vi "eDIDS-24XX-FPGA2-EPTx.vi"() -> ()   [LabVIEW 2015, in "ECS-FPGA.lvlib"]
uses:
  ECS-FPGA.lvlib
  <vilib>/Powertrain Controls/Device Drivers/Engine Position Tracking/EPTx/RevA/FPGA/Controls/EPTxTooth.ctl
  <vilib>/Powertrain Controls/Device Drivers/Engine Position Tracking/EPTx/RevA/FPGA/Controls/EPTxControl.ctl
  <vilib>/Powertrain Controls/Device Drivers/Engine Position Tracking/EPTx/RevA/FPGA/Controls/EPTxConfig.ctl
  <vilib>/Powertrain Controls/Device Drivers/Engine Position Tracking/EPTx/RevA/FPGA/Controls/EPTxSupervisor.ctl
  <vilib>/Powertrain Controls/Device Drivers/Engine Position Tracking/EPTx/RevA/FPGA/Controls/EPTxFuelSparkControl.ctl
  <vilib>/Platform/TimedLoop/XDataNode/timing_clust.ctl
  <vilib>/Platform/TimedLoop/XDataNode/nitl_modes.ctl
  <vilib>/Platform/TimedLoop/XDataNode/wakeup.ctl
  <vilib>/Powertrain Controls/Device Drivers/Engine Position Tracking/EPTx/RevA/FPGA/Controls/EPTxSignals.ctl
  <vilib>/rvi/Emulation/niFpgaSctlEmulationGetInTimedLoop.vi
  <vilib>/rvi/Emulation/niFpgaEmulationReportErrorSimple.vi
  <vilib>/rvi/Emulation/niFpgaGetClockAttributes.vi
  <vilib>/rvi/Emulation/niFpgaCriticalErrorInLSC.vi
  <vilib>/rvi/eio/common/nirviEmuTemplateMethod_errors.vi
  <vilib>/Platform/TimedLoop/XDataNode/XDataNode.xnode
  <vilib>/eio/EIONode/EIONode.xnode
  <vilib>/Platform/TimedLoop/XDataNode/XDNodeRunTimeDep.lvlib
  <vilib>/Powertrain Controls/Device Drivers/Engine Position Tracking/EPTx/RevA/FPGA/EPTx - RevA - FPGA.lvlib
panel:
  out "O2-1.Data":T1
  in  "O2-1.Control":T2
  in  "ESTTL-2.Sequences":T3(array[cluster])
  in  "ESTTL-2.Config":T4
  in  "ESTTL-1.Config":T4
  in  "ESTTL-1.Sequences":T3(array[cluster])
  in  "PFI-1.FuelControl 4":T5
  in  "PFI-1.FuelControl 3":T5
  in  "PFI-1.FuelControl 2":T5
  in  "PFI-1.FuelControl 1":T5
  out "PFI-1.Data":T6 caption="PFIData"
  in  "PFI-1.IPhaseInterface":T7(array[cluster])=[{"IPhaseCurrent"=0, "IPhaseDuration"=0}, {"IPhaseCurrent"=0, "IPhaseDuration"=0}, {"IPhaseCurrent"=0, "IPhaseDuration"=0}, {"IPhaseCurrent"=0, "IPhaseDuration"=0}, {"IPhaseCurrent"=0, "IPhaseDuration"=0}, {"IPhaseCurrent"=0, "IPhaseDuration"=0}, {"IPhaseCurrent"=0, "IPhaseDuration"=0}, {"IPhaseCurrent"=0, "IPhaseDuration"=0}] caption="IPhaseInterface"
  in  "PFI-1.LowsidePWM":T8 caption="LowsidePWM"
  in  "PFI-1.Control":T9 caption="PFIControl"
  in  "PFI-2.Control":T9 caption="PFIControl"
  in  "PFI-2.LowsidePWM":T8 caption="LowsidePWM"
  in  "PFI-2.IPhaseInterface":T7(array[cluster])=[{"IPhaseCurrent"=0, "IPhaseDuration"=0}, {"IPhaseCurrent"=0, "IPhaseDuration"=0}, {"IPhaseCurrent"=0, "IPhaseDuration"=0}, {"IPhaseCurrent"=0, "IPhaseDuration"=0}, {"IPhaseCurrent"=0, "IPhaseDuration"=0}, {"IPhaseCurrent"=0, "IPhaseDuration"=0}, {"IPhaseCurrent"=0, "IPhaseDuration"=0}, {"IPhaseCurrent"=0, "IPhaseDuration"=0}] caption="IPhaseInterface"
  out "PFI-2.Data":T6 caption="PFIData"
  in  "PFI-2.FuelControl 1":T5
  in  "PFI-2.FuelControl 2":T5
  in  "PFI-2.FuelControl 3":T5
  in  "PFI-2.FuelControl 4":T5
  in  "EPTx.Aux3":u8
  in  "EPTx.Primary":u8
  in  "EPTx.Aux1":u8
  out "EPTxSupervisor":T10
  in  "EPTxConfig":T11
  in  "EPTxControl":T12
  out "EPTxTooth":T13
  in  "EPTx.Aux2":u8
  in  "EPTx.Aux4":u8
  out "VRHall-1.DigitalTriggers":u32
  out "Throttle-1.Data":T14 caption="ThrottleData"
  in  "Throttle-1.Control":T15 caption="ThrottleControl"
  out "9411-3.5.PPWData":T16
  out "9411-3.4.PPWData":T16
  out "9411-3.3.PPWData":T16
  out "9411-3.2.PPWData":T16
  out "9411-3.1.PPWData":T16
  out "9411-3.0.PPWData":T16
  in  "9411-3.0.Filt":u16
  in  "9411-3.1.Filt":u16
  in  "9411-3.2.Filt":u16
  in  "9411-3.3.Filt":u16
  in  "9411-3.4.Filt":u16
  in  "9411-3.5.Filt":u16
  in  "9411-3.Invert":u8
  out "9411-3.DigitalTriggers":u32
  out "VRHall-1.6.PPWData":T16
  out "VRHall-1.5.PPWData":T16
  out "VRHall-1.4.PPWData":T16
  out "VRHall-1.3.PPWData":T16
  out "VRHall-1.2.PPWData":T16
  out "VRHall-1.1.PPWData":T16
  in  "VRHall-1.Invert":u8
  in  "VRHall-1.5.Filt":u16
  in  "VRHall-1.4.Filt":u16
  in  "VRHall-1.3.Filt":u16
  in  "VRHall-1.2.Filt":u16
  in  "VRHall-1.1.Filt":u16
  in  "VRHall-1.6.Filt":u16
  out "VRHall-1.Data":T17 caption="VrHallData"
  in  "VRHall-1.Control":T18 caption="VrHallControl"
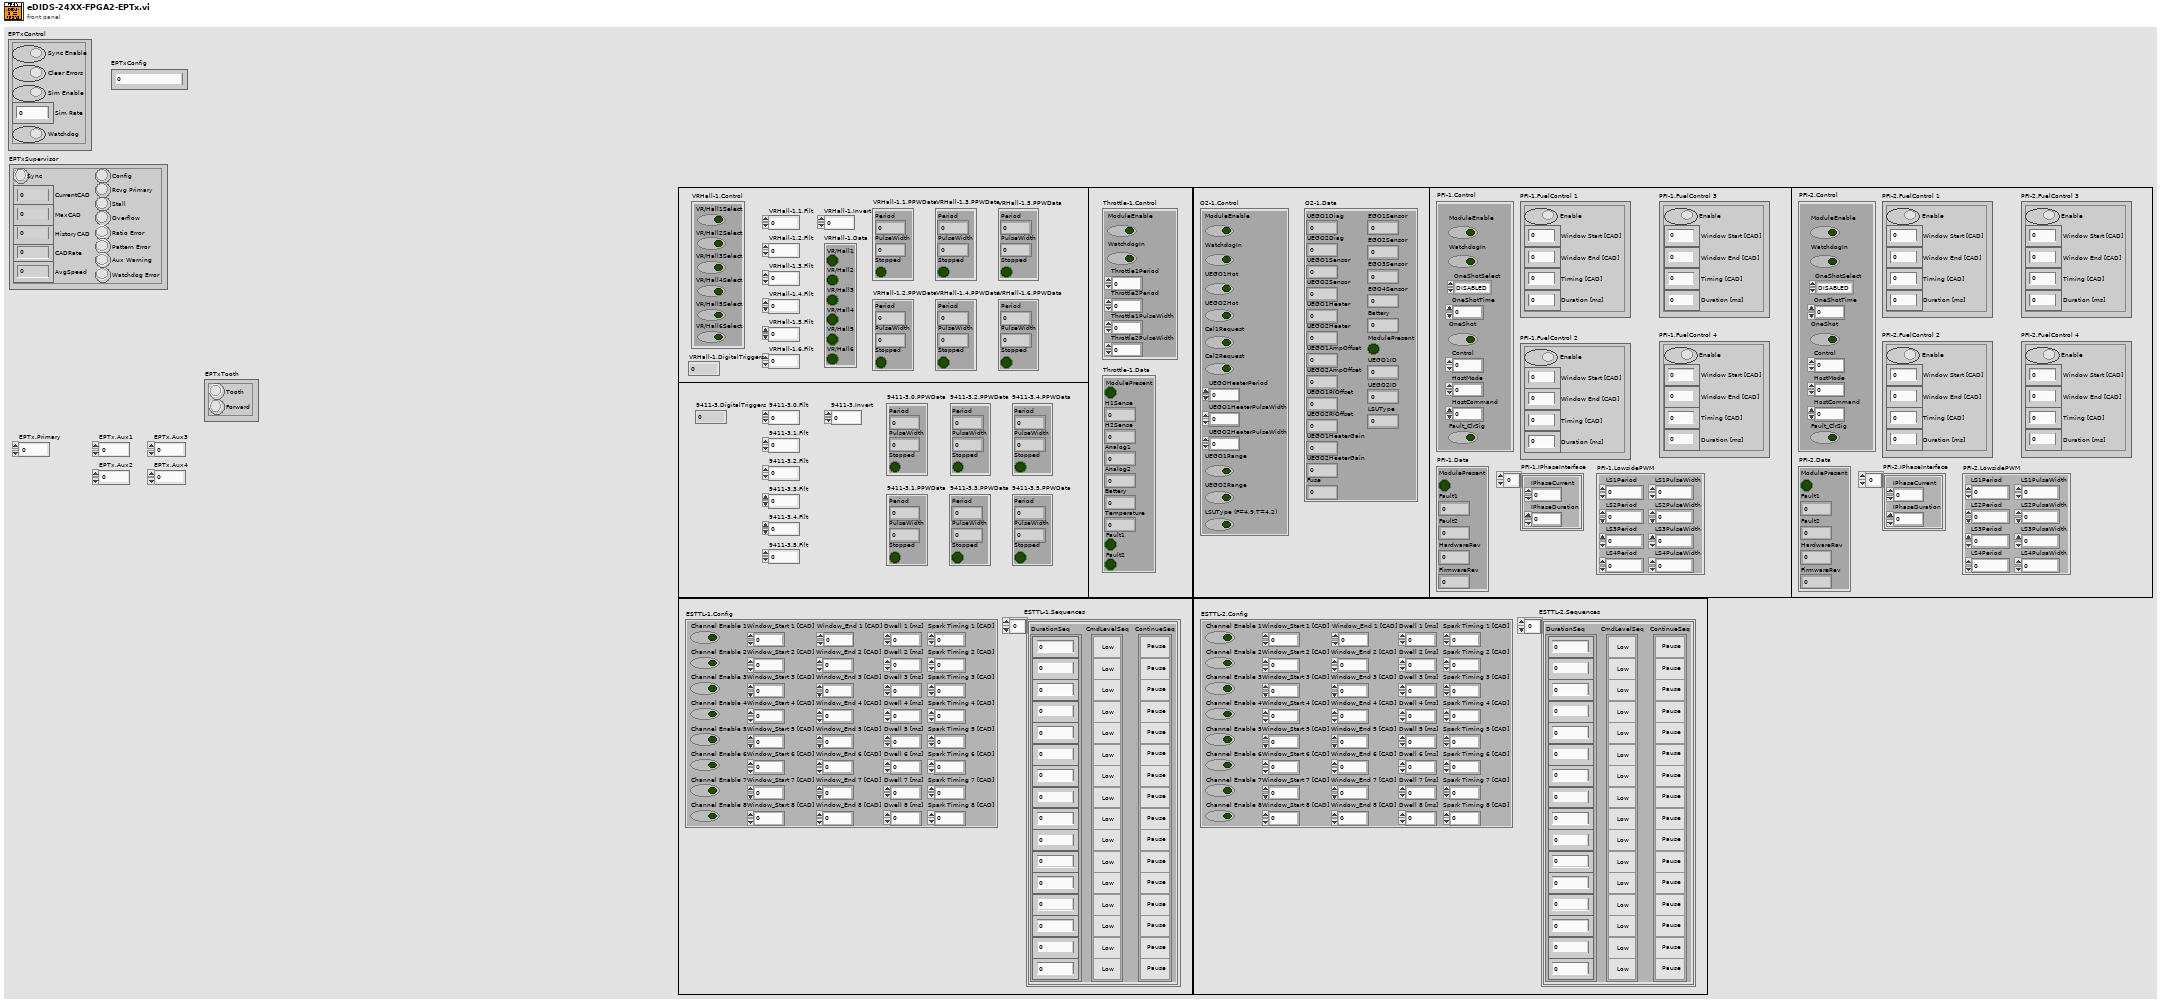
[diagram p1: front panel]
types:
  T1 = cluster{"UEGO1Diag":u8, "UEGO2Diag":u8, "UEGO1Sensor":u16, "UEGO2Sensor":u16, "UEGO1Heater":u16, "UEGO2Heater":u16, "UEGO1AmpOffset":u16, "UEGO2AmpOffset":u16, "UEGO1RIOffset":u16, "UEGO2RIOffset":u16, "UEGO1HeaterGain":u16, "UEGO2HeaterGain":u16, "Fuse":u16, "EGO1Sensor":u16, "EGO2Sensor":u16, "EGO3Sensor":u16, "EGO4Sensor":u16, "Battery":u16, "ModulePresent":bool, "UEGO1ID":u8, "UEGO2ID":u8, "LSUType":u8}
  T2 = cluster{"ModuleEnable":bool, "WatchdogIn":bool, "UEGO1Hot":bool, "UEGO2Hot":bool, "Cal1Request":bool, "Cal2Request":bool, "UEGOHeaterPeriod":u16, "UEGO1HeaterPulseWidth":u16, "UEGO2HeaterPulseWidth":u16, "UEGO1Range":bool, "UEGO2Range":bool, "LSUType (F=4.9,T=4.2)":bool}
  T3 = cluster{"DurationSeq":u32[], "CmdLevelSeq":bool[], "ContinueSeq":bool[]}[]
  T4 = cluster{"Channel Enable 1":bool, "Window_Start 1 [CAD]":fxp<+,18,11>, "Window_End 1 [CAD]":fxp<+,18,11>, "Dwell 1 [ms]":fxp<+/-,22,9>, "Spark Timing 1 [CAD]":fxp<+,18,11>, "Channel Enable 2":bool, "Window_Start 2 [CAD]":fxp<+,18,11>, "Window_End 2 [CAD]":fxp<+,18,11>, "Dwell 2 [ms]":fxp<+/-,22,9>, "Spark Timing 2 [CAD]":fxp<+,18,11>, "Channel Enable 3":bool, "Window_Start 3 [CAD]":fxp<+,18,11>, "Window_End 3 [CAD]":fxp<+,18,11>, "Dwell 3 [ms]":fxp<+/-,22,9>, "Spark Timing 3 [CAD]":fxp<+,18,11>, "Channel Enable 4":bool, "Window_Start 4 [CAD]":fxp<+,18,11>, "Window_End 4 [CAD]":fxp<+,18,11>, "Dwell 4 [ms]":fxp<+/-,22,9>, "Spark Timing 4 [CAD]":fxp<+,18,11>, "Channel Enable 5":bool, "Window_Start 5 [CAD]":fxp<+,18,11>, "Window_End 5 [CAD]":fxp<+,18,11>, "Dwell 5 [ms]":fxp<+/-,22,9>, "Spark Timing 5 [CAD]":fxp<+,18,11>, "Channel Enable 6":bool, "Window_Start 6 [CAD]":fxp<+,18,11>, "Window_End 6 [CAD]":fxp<+,18,11>, "Dwell 6 [ms]":fxp<+/-,22,9>, "Spark Timing 6 [CAD]":fxp<+,18,11>, "Channel Enable 7":bool, "Window_Start 7 [CAD]":fxp<+,18,11>, "Window_End 7 [CAD]":fxp<+,18,11>, "Dwell 7 [ms]":fxp<+/-,22,9>, "Spark Timing 7 [CAD]":fxp<+,18,11>, "Channel Enable 8":bool, "Window_Start 8 [CAD]":fxp<+,18,11>, "Window_End 8 [CAD]":fxp<+,18,11>, "Dwell 8 [ms]":fxp<+/-,22,9>, "Spark Timing 8 [CAD]":fxp<+,18,11>}
  T5 = typedef "EPTx - RevA - FPGA.lvlib/EPTxFuelSparkControl.ctl" = cluster{"Enable":bool, "Window Start [CAD]":fxp<+,18,11>, "Window End [CAD]":fxp<+,18,11>, "Timing [CAD]":fxp<+,18,11>, "Duration [ms]":fxp<+/-,22,9>}
  T6 = cluster{"ModulePresent":bool, "Fault1":u8, "Fault2":u8, "HardwareRev":u8, "FirmwareRev":u8}
  T7 = cluster{"IPhaseCurrent":u16, "IPhaseDuration":u16}[]
  T8 = cluster{"LS1Period":u32, "LS1PulseWidth":u32, "LS2Period":u32, "LS2PulseWidth":u32, "LS3Period":u32, "LS3PulseWidth":u32, "LS4Period":u32, "LS4PulseWidth":u32}
  T9 = cluster{"ModuleEnable":bool, "WatchdogIn":bool, "OneShotSelect":enum8{"DISABLED", "PFI 1", "PFI 2", "PFI 3", "PFI 4"}, "OneShotTime":u32, "OneShot":bool, "Control":u16, "HostMode":u8, "HostCommand":u32, "Fault_ClrSig":bool}
  T10 = typedef "EPTx - RevA - FPGA.lvlib/EPTxSupervisor.ctl" = cluster{"Sync":bool, "CurrentCAD":fxp<+,18,11>, "MaxCAD":fxp<+,11,11>, "HistoryCAD":fxp<+,11,11>, "CADRate":fxp<+,22,8>, "AvgSpeed":fxp<+,17,15>, "Config":bool, "Rcvg Primary":bool, "Stall":bool, "Overflow":bool, "Ratio Error":bool, "Pattern Error":bool, "Aux Warning":bool, "Watchdog Error":bool}
  T11 = typedef "EPTx - RevA - FPGA.lvlib/EPTxConfig.ctl" = u64
  T12 = typedef "EPTx - RevA - FPGA.lvlib/EPTxControl.ctl" = cluster{"Sync Enable":bool, "Clear Errors":bool, "Sim Enable":bool, "Sim Rate":fxp<+,24,6>, "Watchdog":bool}
  T13 = typedef "EPTx - RevA - FPGA.lvlib/EPTxTooth.ctl" = cluster{"Tooth":bool, "Forward":bool}
  T14 = cluster{"ModulePresent":bool, "H1Sense":i16, "H2Sense":i16, "Analog1":i16, "Analog2":i16, "Battery":i16, "Temperature":i16, "Fault1":bool, "Fault2":bool}
  T15 = cluster{"ModuleEnable":bool, "WatchdogIn":bool, "Throttle1Period":u16, "Throttle2Period":u16, "Throttle1PulseWidth":i16, "Throttle2PulseWidth":i16}
  T16 = cluster{"Period":u32, "PulseWidth":u32, "Stopped":bool}
  T17 = cluster{"VR/Hall1":bool, "VR/Hall2":bool, "VR/Hall3":bool, "VR/Hall4":bool, "VR/Hall5":bool, "VR/Hall6":bool}
  T18 = cluster{"VR/Hall1Select":bool, "VR/Hall2Select":bool, "VR/Hall3Select":bool, "VR/Hall4Select":bool, "VR/Hall5Select":bool, "VR/Hall6Select":bool}
  T19 = typedef "XDNodeRunTimeDep.lvlib/timing_clust.ctl" = cluster{"Expected End [f-1]":u64, "Actual End [f-1]":u64, "Finished Late? [f-1]":bool, "Expected End [i-1]":u64, "Actual End [i-1]":u64, "Finished Late? [i-1]":bool, "Expected Start [i]":u64, "Actual Start [i]":u64, "Expected Start [f]":u64, "Actual Start [f]":u64, "Source Name":string, "Structure Name":string, "Period":i64, "Deadline":i64, "Offset":i64, "Start":i64, "Priority":i32, "Timeout":i32, "Mode":T20, "Wakeup Reason":T21, "Error":errorcluster, "Source Type":string, "Secondary Source Type":string, "Global End Time":u64, "Global Start Time":u64, "Frame Duration":u64, "Iteration Duration":u64, "Assigned CPU":i32, "I/O Scan Engine Mode":u32}
  T20 = typedef "XDNodeRunTimeDep.lvlib/nitl_modes.ctl" = enum32{"No Change", "Process missed periods, maintain original phase", "Discard missed periods, maintain original phase", "Process missed periods, ignore original phase", "Discard missed periods, ignore original phase"}
  T21 = typedef "XDNodeRunTimeDep.lvlib/wakeup.ctl" = enum32{"Normal", "Aborted", "Asynchronous wakeup", "Timing source error", "Timed loop error", "Timeout"}
  T22 = typedef "EPTx - RevA - FPGA.lvlib/EPTxSignals.ctl" = cluster{"Primary":bool, "Aux 1":bool, "Aux 2":bool, "Aux 3":bool, "Aux 4":bool}
  T23 = cluster{"9411-3.0.Filt":u16, "9411-3.1.Filt":u16, "9411-3.2.Filt":u16, "9411-3.3.Filt":u16, "9411-3.4.Filt":u16, "9411-3.5.Filt":u16}
  T24 = cluster{"VRHall-1.1.Filt":u16, "VRHall-1.2.Filt":u16, "VRHall-1.3.Filt":u16, "VRHall-1.4.Filt":u16, "VRHall-1.5.Filt":u16, "VRHall-1.6.Filt":u16}
  T25 = cluster{"CmdOut1":bool, "CmdOut2":bool, "CmdOut3":bool, "CmdOut4":bool, "CmdOut5":bool, "CmdOut6":bool, "CmdOut7":bool, "CmdOut8":bool}
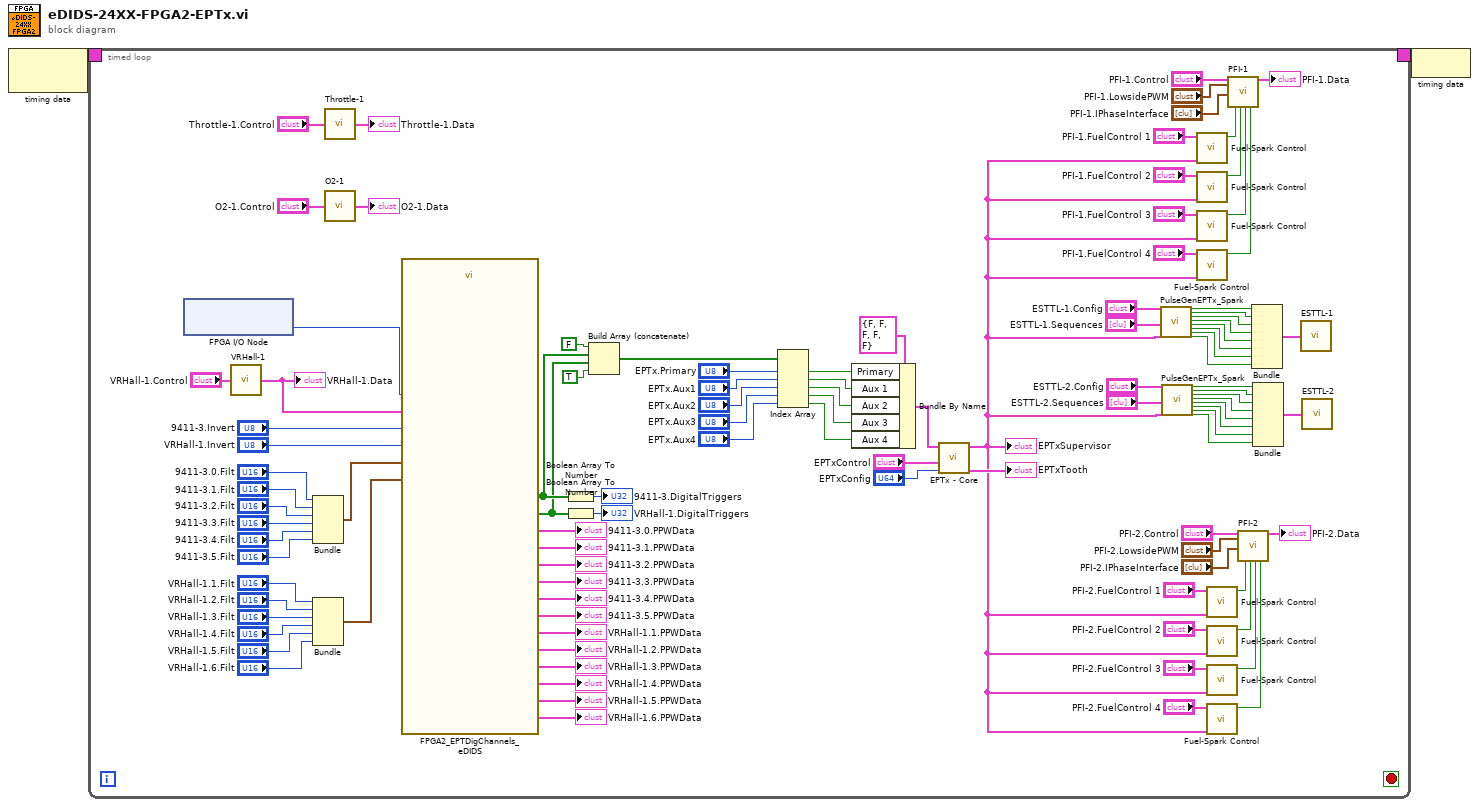
[diagram p0: block diagram]
diagram:
  n1 = node-c288() -> (w2:T19)  [unwired: 1 in]
  n2 = timed-loop {
    timing: w2 -> [_]
    timing-out: [_] -> w1
    stop <- _ stop-if-true
    n3 = xnode "FPGA I/O Node"() -> ("9411-3/DI5:0"=w89:u8)  [unwired: 1 in, 1 out]
    n4 = call "VRHall-1"("VRHall-1_Control"="VRHall-1.Control") -> ("VRHall-1_Data"=w90:T17)
    "VRHall-1.Data" <- w90
    n5 = Bundle("9411-3.0.Filt"="9411-3.0.Filt", "9411-3.1.Filt"="9411-3.1.Filt", "9411-3.2.Filt"="9411-3.2.Filt", "9411-3.3.Filt"="9411-3.3.Filt", "9411-3.4.Filt"="9411-3.4.Filt", "9411-3.5.Filt"="9411-3.5.Filt") -> (w82:T23)  [unwired: 1 in]
    n6 = Bundle("VRHall-1.1.Filt"="VRHall-1.1.Filt", "VRHall-1.2.Filt"="VRHall-1.2.Filt", "VRHall-1.3.Filt"="VRHall-1.3.Filt", "VRHall-1.4.Filt"="VRHall-1.4.Filt", "VRHall-1.5.Filt"="VRHall-1.5.Filt", "VRHall-1.6.Filt"="VRHall-1.6.Filt") -> (w92:T24)  [unwired: 1 in]
    n7 = call "Throttle-1"("Throttle-1_Control"="Throttle-1.Control") -> ("Throttle-1_Data"=→"Throttle-1.Data":T14)
    n8 = call "O2-1"("O2Control"="O2-1.Control") -> ("O2Data"=→"O2-1.Data":T1)
    n9 = call "FPGA2_EPTDigChannels_eDIDS.vi"("NI 9411-3/DI5:0"=w89, "VRHall-1.Data"=w90, "9411-3.Invert"="9411-3.Invert", "VRHall-1.Invert"="VRHall-1.Invert", "9411-3.FilterValues"=w82, "VRHall-1.FilterValues"=w92) -> ("9411-3.0.PPWData"=→"9411-3.0.PPWData":T16, "VRHall-1.1.PPWData"=→"VRHall-1.1.PPWData":T16, "9411-3.1.PPWData"=→"9411-3.1.PPWData":T16, "VRHall-1.2.PPWData"=→"VRHall-1.2.PPWData":T16, "9411-3.2.PPWData"=→"9411-3.2.PPWData":T16, "VRHall-1.3.PPWData"=→"VRHall-1.3.PPWData":T16, "9411-3.3.PPWData"=→"9411-3.3.PPWData":T16, "VRHall-1.4.PPWData"=→"VRHall-1.4.PPWData":T16, "9411-3.4.PPWData"=→"9411-3.4.PPWData":T16, "VRHall-1.5.PPWData"=→"VRHall-1.5.PPWData":T16, "9411-3.5.PPWData"=→"9411-3.5.PPWData":T16, "VRHall-1.6.PPWData"=→"VRHall-1.6.PPWData":T16, "9411-3.DigitalTriggers"=w72:bool[], "VRHall-1.DigitalTriggers"=w71:bool[])  [unwired: 8 in]
    n10 = Boolean Array To Number(Boolean array=w72) -> (number=→"9411-3.DigitalTriggers":u32)
    n11 = Boolean Array To Number(Boolean array=w71) -> (number=→"VRHall-1.DigitalTriggers":u32)
    n12 = Build Array (concatenate)(FALSE, w72, w71, TRUE) -> (w52:bool[])
    n13 = Index Array(array=w52, index #1="EPTx.Primary", index #2="EPTx.Aux1", index #3="EPTx.Aux2", index #4="EPTx.Aux3", index #5="EPTx.Aux4") -> (element #1=w61:bool, element #2=w62:bool, element #3=w63:bool, element #4=w64:bool, element #5=w65:bool)
    n14 = Bundle By Name(cluster=T22 {"Primary"=FALSE, "Aux 1"=FALSE, "Aux 2"=FALSE, "Aux 3"=FALSE, "Aux 4"=FALSE} ("EPTxSignals"), "Primary"=w61, "Aux 1"=w62, "Aux 2"=w63, "Aux 3"=w64, "Aux 4"=w65) -> (w54:T22)
    n15 = call <vilib>:"EPTx - Core.vi"("EPTxConfig"="EPTxConfig", "EPTxControl"="EPTxControl", "EPTxSignals"=w54) -> ("EPTxTooth"=→"EPTxTooth":T13, "EPTxSupervisor"=w5:T10)  [unwired: 7 in]
    "EPTxSupervisor" <- w5
    n16 = call "PulseGenEPTx_Spark.vi"("Spark_Config"="ESTTL-1.Config", "Spark_Sequences"="ESTTL-1.Sequences", "EPTxSupervisor"=w5) -> ("CmdOut1"=w17:bool, "CmdOut2"=w18:bool, "CmdOut3"=w19:bool, "CmdOut4"=w20:bool, "CmdOut5"=w21:bool, "CmdOut6"=w22:bool, "CmdOut7"=w23:bool, "CmdOut8"=w24:bool)  [unwired: 17 in]
    n17 = call "PulseGenEPTx_Spark.vi"("Spark_Config"="ESTTL-2.Config", "Spark_Sequences"="ESTTL-2.Sequences", "EPTxSupervisor"=w5) -> ("CmdOut1"=w16:bool, "CmdOut2"=w15:bool, "CmdOut3"=w14:bool, "CmdOut4"=w13:bool, "CmdOut5"=w12:bool, "CmdOut6"=w11:bool, "CmdOut7"=w10:bool, "CmdOut8"=w9:bool)  [unwired: 17 in]
    n18 = call <vilib>:"Fuel-Spark Control.vi"("EPTxSupervisor"=w5, "Fuel-Spark Control"="PFI-1.FuelControl 1") -> ("Fuel-Spark Command"=w28:bool)  [unwired: 9 in]
    n19 = call <vilib>:"Fuel-Spark Control.vi"("EPTxSupervisor"=w5, "Fuel-Spark Control"="PFI-1.FuelControl 2") -> ("Fuel-Spark Command"=w29:bool)  [unwired: 9 in]
    n20 = call <vilib>:"Fuel-Spark Control.vi"("EPTxSupervisor"=w5, "Fuel-Spark Control"="PFI-1.FuelControl 3") -> ("Fuel-Spark Command"=w30:bool)  [unwired: 9 in]
    n21 = call <vilib>:"Fuel-Spark Control.vi"("EPTxSupervisor"=w5, "Fuel-Spark Control"="PFI-1.FuelControl 4") -> ("Fuel-Spark Command"=w31:bool)  [unwired: 9 in]
    n22 = call <vilib>:"Fuel-Spark Control.vi"("EPTxSupervisor"=w5, "Fuel-Spark Control"="PFI-2.FuelControl 1") -> ("Fuel-Spark Command"=w51:bool)  [unwired: 9 in]
    n23 = call <vilib>:"Fuel-Spark Control.vi"("EPTxSupervisor"=w5, "Fuel-Spark Control"="PFI-2.FuelControl 2") -> ("Fuel-Spark Command"=w50:bool)  [unwired: 9 in]
    n24 = call <vilib>:"Fuel-Spark Control.vi"("EPTxSupervisor"=w5, "Fuel-Spark Control"="PFI-2.FuelControl 3") -> ("Fuel-Spark Command"=w49:bool)  [unwired: 9 in]
    n25 = call <vilib>:"Fuel-Spark Control.vi"("EPTxSupervisor"=w5, "Fuel-Spark Control"="PFI-2.FuelControl 4") -> ("Fuel-Spark Command"=w48:bool)  [unwired: 9 in]
    n26 = call "PFI-1"("PFI-1_Control"="PFI-1.Control", "PFI-1_LowsidePWM"="PFI-1.LowsidePWM", "PFI-1_IPhaseInterface"="PFI-1.IPhaseInterface", "PFI1Cmd"=w28, "PFI2Cmd"=w29, "PFI3Cmd"=w30, "PFI4Cmd"=w31) -> ("PFI-1_Data"=→"PFI-1.Data":T6)  [unwired: 11 in, 1 out]
    n27 = call "PFI-2"("PFI-2_Control"="PFI-2.Control", "PFI-2_LowsidePWM"="PFI-2.LowsidePWM", "PFI-2_IPhaseInterface"="PFI-2.IPhaseInterface", "PFI1Cmd"=w51, "PFI2Cmd"=w50, "PFI3Cmd"=w49, "PFI4Cmd"=w48) -> ("PFI-2_Data"=→"PFI-2.Data":T6)  [unwired: 11 in, 1 out]
    n28 = Bundle("CmdOut1"=w17, "CmdOut2"=w18, "CmdOut3"=w19, "CmdOut4"=w20, "CmdOut5"=w21, "CmdOut6"=w22, "CmdOut7"=w23, "CmdOut8"=w24) -> (w25:T25)  [unwired: 1 out]
    n29 = Bundle("CmdOut1"=w16, "CmdOut2"=w15, "CmdOut3"=w14, "CmdOut4"=w13, "CmdOut5"=w12, "CmdOut6"=w11, "CmdOut7"=w10, "CmdOut8"=w9) -> (w8:T25)  [unwired: 1 out]
    n30 = call "ESTTL-1"("ESTTL-1_ESTTLChan"=w25) -> ()  [unwired: 1 out]
    n31 = call "ESTTL-2"("ESTTL-2_ESTTLChan"=w8) -> ()  [unwired: 1 out]
  }
  n32 = node-c288(w1) -> ()
